vi "SolarControl.vi"(7 "Timer State In":T1, 8 "Error In":errorcluster, 9 "FPGA Data In":T2, 10 "ES System Data In":T3={"Voltage"=0.0, "Current"=0.0, "SOC Avg"=0.0, "Faults"=0, "Alarms"=0, "Number of Strings"=0, "Max Temp"=0, "Min Temp"=0, "Max Cell Voltage"=0.0, "Min Cell Voltage"=0.0, "Energy Capacity (kWh)"=0.0, "Energy Remaining (kWh)"=0.0, "SOC Min"=0.0, "SOC Max"=0.0, "ES Fault"=FALSE, "String Selector"=enum."3 Strings"}, 11 "State":T5) -> (0 "Error Out":errorcluster, 3 "PV Control":bool, 5 "Timer State Out":T1={"Start Time"=0, "Timer State"=enum."Start Timer"})   [LabVIEW 2013]
uses:
  eng/trunk/ni/cRIO Master Files/Controls/RTStateMachine.ctl
  eng/trunk/ni/cRIO Master Files/Controls/EnergyStorageSystemData.ctl
  eng/trunk/ni/cRIO Master Files/Controls/StringSelector.ctl
  Controls/FPGAData.ctl
  eng/trunk/ni/cRIO Master Files/Controls/TimerData.ctl
  <vilib>/ptbypt/NI_PtbyPt.lvlib
panel:
  in  "PV":bool
  in  "Solar Gen":sgl
  in  "Solar SSG":sgl
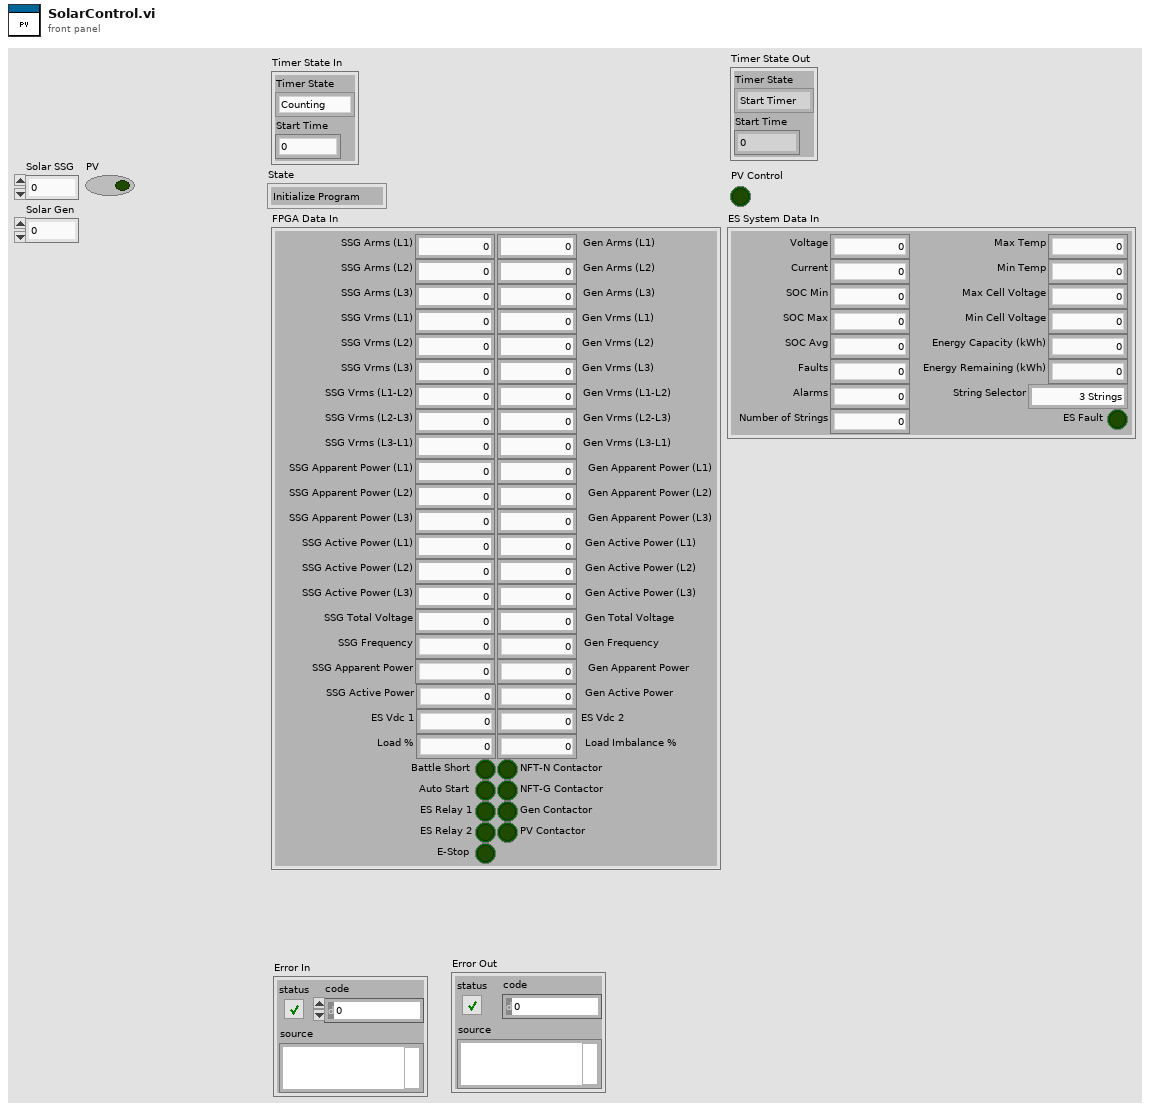
[diagram p1: front panel]
types:
  T1 = typedef "TimerData.ctl" = cluster{"Start Time":u32, "Timer State":enum16{"Counting", "Start Timer"}}
  T2 = typedef "FPGAData.ctl" = cluster{"SSG Frequency":sgl, "SSG Total Voltage":dbl, "SSG Active Power":sgl, "SSG Apparent Power":sgl, "SSG Active Power (L1)":dbl, "SSG Active Power (L2)":dbl, "SSG Active Power (L3)":dbl, "SSG Apparent Power (L1)":dbl, "SSG Apparent Power (L2)":dbl, "SSG Apparent Power (L3)":dbl, "SSG Vrms (L1-L2)":dbl, "SSG Vrms (L2-L3)":dbl, "SSG Vrms (L3-L1)":dbl, "SSG Vrms (L1)":dbl, "SSG Vrms (L2)":dbl, "SSG Vrms (L3)":dbl, "SSG Arms (L1)":dbl, "SSG Arms (L2)":dbl, "SSG Arms (L3)":dbl, "Gen Frequency":sgl, "Gen Total Voltage":dbl, "Gen Active Power":sgl, "Gen Apparent Power":sgl, "Gen Active Power (L1)":dbl, "Gen Active Power (L2)":dbl, "Gen Active Power (L3)":dbl, "Gen Apparent Power (L1)":dbl, "Gen Apparent Power (L2)":dbl, "Gen Apparent Power (L3)":dbl, "Gen Vrms (L1-L2)":dbl, "Gen Vrms (L2-L3)":dbl, "Gen Vrms (L3-L1)":dbl, "Gen Vrms (L1)":dbl, "Gen Vrms (L2)":dbl, "Gen Vrms (L3)":dbl, "Gen Arms (L1)":dbl, "Gen Arms (L2)":dbl, "Gen Arms (L3)":dbl, "ES Vdc 1":sgl, "ES Vdc 2":sgl, "Load %":sgl, "Load Imbalance %":sgl, "E-Stop":bool, "Battle Short":bool, "Auto Start":bool, "Gen Contactor":bool, "ES Relay 1":bool, "ES Relay 2":bool, "NFT-N Contactor":bool, "NFT-G Contactor ":bool, "PV Contactor":bool}
  T3 = typedef "EnergyStorageSystemData.ctl" = cluster{"Voltage":sgl, "Current":sgl, "SOC Avg":sgl, "Faults":u16, "Alarms":u16, "Number of Strings":u16, "Max Temp":i16, "Min Temp":i16, "Max Cell Voltage":sgl, "Min Cell Voltage":sgl, "Energy Capacity (kWh)":sgl, "Energy Remaining (kWh)":sgl, "SOC Min":sgl, "SOC Max":sgl, "ES Fault":bool, "String Selector":T4}
  T4 = typedef "StringSelector.ctl" = enum16{"1 String (1)", "1 String (2)", "1 String (3)", "2 Strings (1, 2)", "2 Strings (2, 3)", "2 Strings (1, 3)", "3 Strings"}
  T5 = typedef "RTStateMachine.ctl" = enum16{"Initialize Program", "Big Boss Startup 1", "Big Boss Startup 2", "Big Boss Startup 3", "Big Boss Startup 4", "Big Boss Startup 5", "Big Boss Startup 6", "Shiner Startup 1", "Shiner Startup 2", "Shiner Startup 3", "Shiner Startup 4", "Shiner Startup 5", "Shiner Startup 6", "Shiner Startup 7", "Shiner Startup 8", "Shiner Startup 9", "Discharge", "Init Batteries", "Start s120", "enable batteries", "s120 Voltage Match", "Reset Batteries", "Wait for Event", "System Standby", "StandbyToRunning", "System Running", "SSG Enabled", "SpotGen Start", "SpotGen Charge", "SpotGen Desync", "SpotGen Discharge", "SpotGen Sync", "Peak Shave", "Charge Control", "Manual Current", "Inhibit Control", "Stop System", "uCap Start 1", "uCap Start 2", "uCap Start 3", "INVALID STATE"}
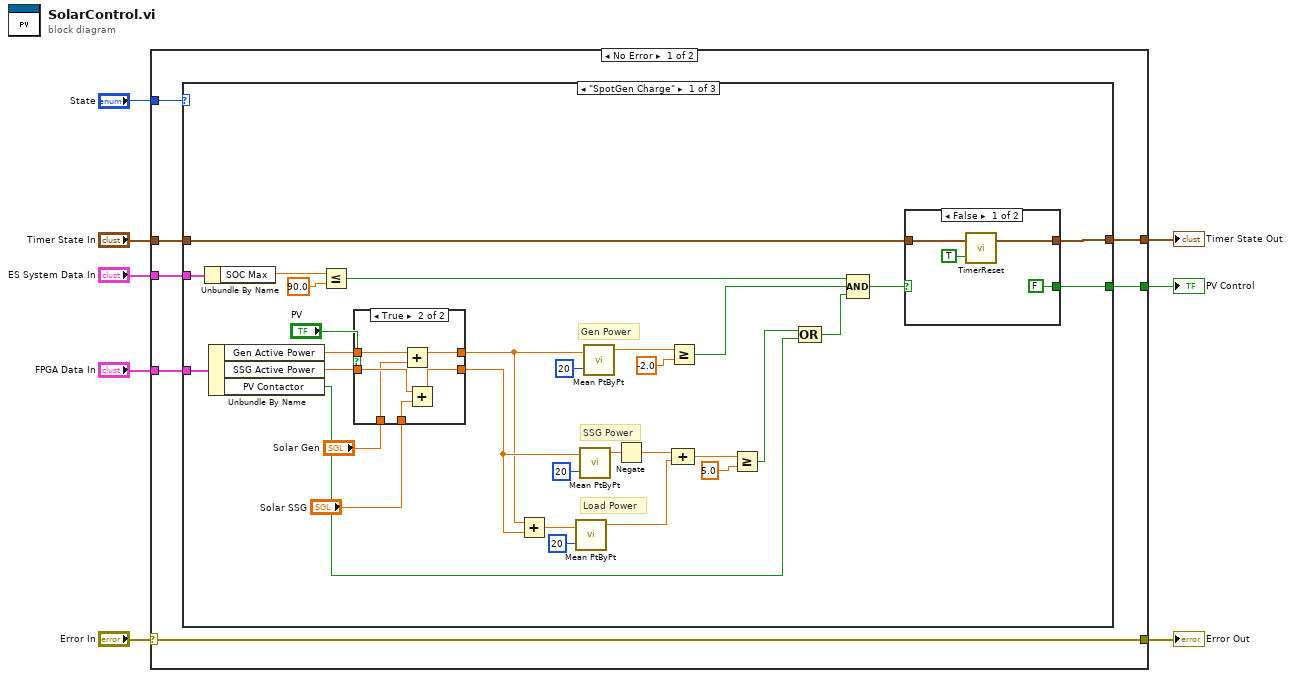
[diagram p0: block diagram]
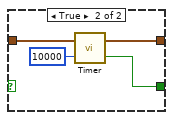
[diagram p3: hidden frame]
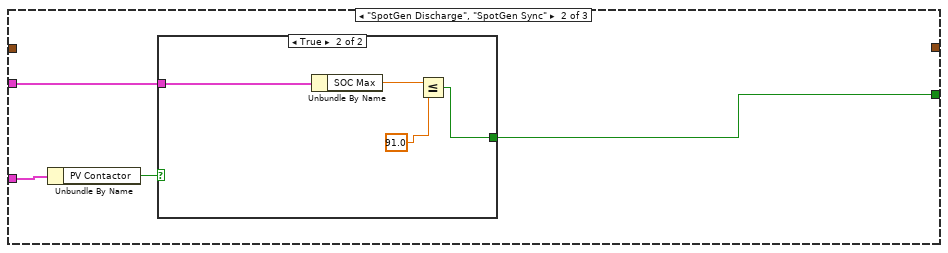
[diagram p4: hidden frame]
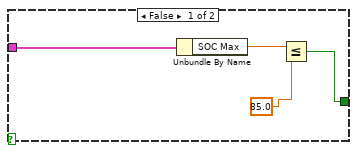
[diagram p5: hidden frame]
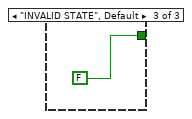
[diagram p6: hidden frame]
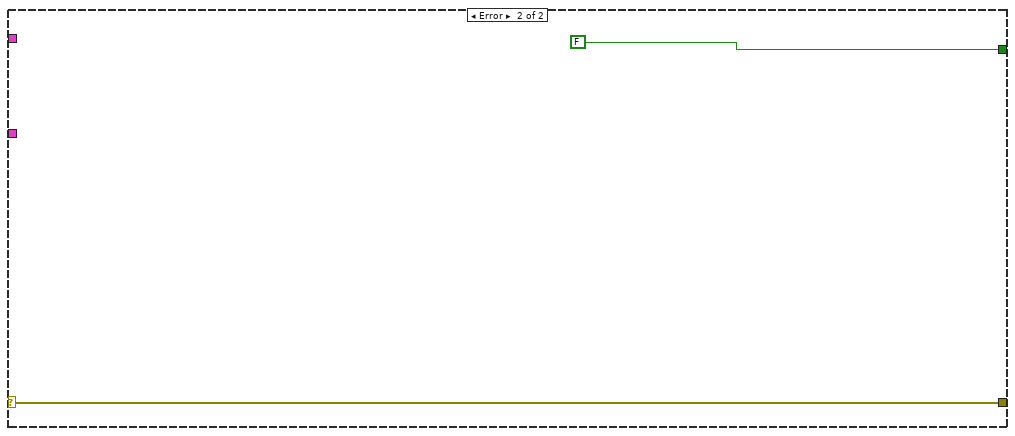
[diagram p7: hidden frame]
diagram:
  n1 = case shown="No Error" "Error In" {
    selector: "Error In" -> [w14 w77]
    tunnel: "State" -> [w15 _]
    tunnel: [w14 w77] -> w6
    tunnel: [w13 FALSE] -> w5
    tunnel: "ES System Data In" -> [w12 _]
    tunnel: "FPGA Data In" -> [w11 _]
    tunnel: "Timer State In" -> [w10 _]
    tunnel: [w9 _] -> w1
    frame No Error {
      n2 = case shown="\"SpotGen Charge\"" w15 {
        tunnel: [w35 w63 FALSE] -> w13
        tunnel: w12 -> [w45 w65 _]
        tunnel: w11 -> [w46 w66 _]
        tunnel: w10 -> [w37 _ _]
        tunnel: [w36 _ _] -> w9
        frame "SpotGen Charge" {
          # "Load Power"
          # "SSG Power"
          # "Gen Power"
          n3 = Unbundle By Name(w45) -> ("SOC Max"=w44:sgl)
          n4 = Unbundle By Name(w46) -> ("Gen Active Power"=w39:sgl, "SSG Active Power"=w20:sgl, "PV Contactor"=w25:bool)
          n5 = Less Or Equal?(x=w44, y=sgl 90.0) -> (x <= y?=w43:bool)
          n6 = case shown="True" "PV" {
            tunnel: w39 -> [w48 w54]
            tunnel: [w47 w53] -> w21
            tunnel: w20 -> [w47 w52]
            tunnel: "Solar SSG" -> [_ w51]
            tunnel: [w48 w50] -> w18
            tunnel: "Solar Gen" -> [_ w49]
            frame False {
            }
            frame True {
              n7 = Add(x=w54, y=w49) -> (x+y=w50:sgl)
              n8 = Add(x=w52, y=w51) -> (x+y=w53:sgl)
            }
          }
          n9 = Add(x=w18, y=w21) -> (x+y=w29:sgl)
          n10 = call <vilib>:"Mean PtByPt.vi"("x"=w29, "sample length"=20) -> ("mean"=w27:dbl)  [unwired: 2 in, 1 out]
          n11 = call <vilib>:"Mean PtByPt.vi"("x"=w21, "sample length"=20) -> ("mean"=w32:dbl)  [unwired: 2 in, 1 out]
          n12 = call <vilib>:"Mean PtByPt.vi"("x"=w18, "sample length"=20) -> ("mean"=w40:dbl)  [unwired: 2 in, 1 out]
          n13 = Negate(x=w32) -> (-x=w28:dbl)
          n14 = Greater Or Equal?(x=w40, y=-2.0) -> (x >= y?=w23:bool)
          n15 = Compound Arithmetic op=ADD(w28, w27) -> (w26:dbl)
          n16 = Greater Or Equal?(x=w26, y=5.0) -> (x >= y?=w24:bool)
          n17 = Compound Arithmetic op=OR(w24, w25) -> (w22:bool)
          n18 = Compound Arithmetic op=AND(w43, w23, w22) -> (w38:bool)
          n19 = case shown="False" w38 {
            tunnel: w37 -> [w58 w62]
            tunnel: [w57 w61] -> w36
            tunnel: [FALSE ("Time Expired") w59] -> w35
            frame False {
              n20 = call "TimerReset.vi"("Reset?"=TRUE, "Timer State In"=w58) -> ("Timer State Out"=w57:T1)  [unwired: 1 in]
            }
            frame True {
              n21 = call "Timer.vi"("Time to count (msec)"=u32 10000, "Timer State In"=w62) -> ("Time Expired"=w59:bool, "Timer State Out"=w61:T1)
            }
          }
        }
        frame "SpotGen Discharge", "SpotGen Sync" {
          n22 = Unbundle By Name(w66) -> ("PV Contactor"=w64:bool)
          n23 = case shown="True" w64 {
            tunnel: w65 -> [w68 w72]
            tunnel: [w67 w71] -> w63
            frame False {
              n24 = Unbundle By Name(w68) -> ("SOC Max"=w69:sgl)
              n25 = Less Or Equal?(x=w69, y=sgl 85.0) -> (x <= y?=w67:bool)
            }
            frame True {
              n26 = Unbundle By Name(w72) -> ("SOC Max"=w73:sgl)
              n27 = Less Or Equal?(x=w73, y=sgl 91.0) -> (x <= y?=w71:bool)
            }
          }
        }
        frame "INVALID STATE", Default {
        }
      }
    }
    frame Error {
    }
  }
  "Error Out" <- w6
  "PV Control" <- w5
  "Timer State Out" <- w1
